vi "SetParam.vi"(8 "error in (no error)":errorcluster caption="entrée d'erreur (pas d'erreur)", 10 "MultiLabelBinarizer":T1, 11 "MultiLabelBinarizer.lvclass":refnum<class "MultiLabelBinarizer.lvclass">) -> (0 "error out":errorcluster caption="sortie d'erreur", 3 "MultiLabelBinarizer.lvclass":refnum<class "MultiLabelBinarizer.lvclass">)   [LabVIEW 2020, in "MultiLabelBinarizer.lvclass"]
doc: "Set Parameters"
uses:
  MultiLabelBinarizer.lvclass
  MultiLabelBinarizer.lvclass/MultiLabelBinarizer.ctl
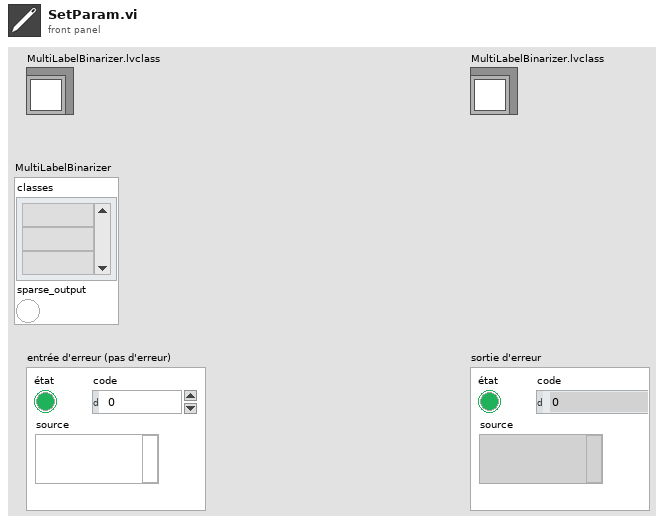
[diagram p1: front panel]
types:
  T1 = cluster{"classes":string[][], "sparse_output":bool}
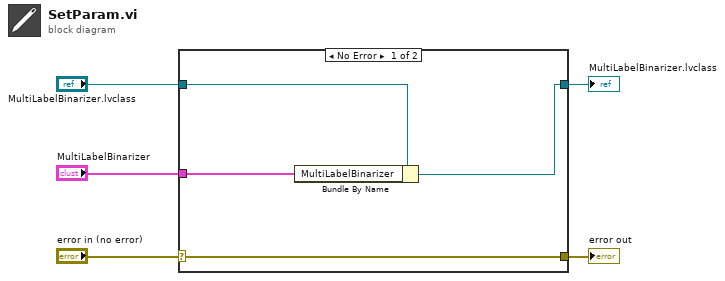
[diagram p0: block diagram]
diagram:
  n1 = case shown="No Error" "error in (no error)" {
    selector: "error in (no error)" -> [w9 w10]
    tunnel: [w9 w10] -> w4
    tunnel: [w7 w11] -> w2
    tunnel: "MultiLabelBinarizer.lvclass" -> [w8 w11]
    tunnel: "MultiLabelBinarizer" -> [w6 _]
    frame No Error {
      n2 = Bundle By Name(cluster=w8, "MultiLabelBinarizer"=w6) -> (w7:refnum<class "MultiLabelBinarizer.lvclass">)
    }
    frame Error {
    }
  }
  "error out" <- w4
  "MultiLabelBinarizer.lvclass" <- w2
